vi "Read Settings File.vi"(11 "FIle_Name":string) -> (2 "HV_Voltage_Number":dbl[](array[numeric]), 3 "HV_Voltage_Value_String":string[](array[string]))   [LabVIEW 2013]
uses:
  <vilib>/Utility/file.llb/Read From Spreadsheet File (string).vi
panel:
  out "HV_Settings":string[](array[string])
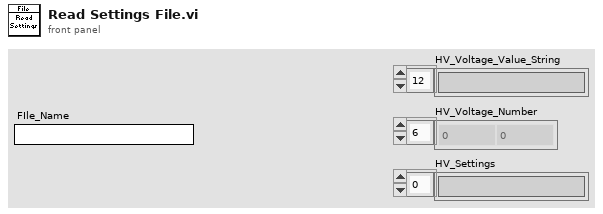
[diagram p1: front panel]
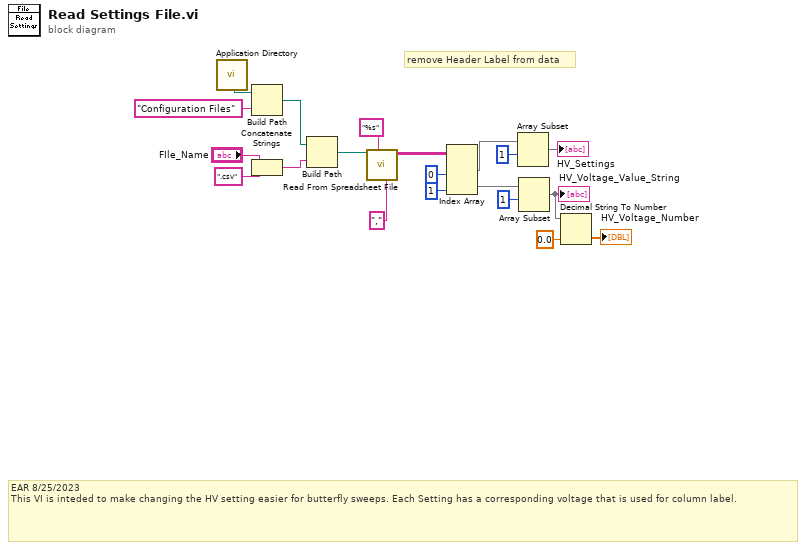
[diagram p0: block diagram]
diagram:
  # "remove Header Label from data"
  # "EAR 8/25/2023\nThis VI is inteded to make changing the HV setting easier for butterfly sweeps. Each Setting has a corresponding voltage that is used for column label."
  n1 = call <vilib>:"Application Directory.vi"() -> ("Application Directory"=w20:path)
  n2 = Build Path(base path=w20, name or relative path="Configuration Files") -> (appended path=w18:path)
  n3 = Concatenate Strings("FIle_Name", ".csv" ("string")) -> (w15:string)
  n4 = Build Path(base path=w18, name or relative path=w15) -> (appended path=w14:path)
  n5 = call-poly <vilib>:"Read From Spreadsheet File.vi"("delimiter (\\t)"="," ("delimiter (\\t)"), "format (%s)"="%s", "file path (dialog if empty)"=w14) -> ("all rows"=w12:string[][])  [unwired: 4 in, 4 out]
  n6 = Index Array(array=w12, index (col) #1=0 ("disabled index (col)"), index (col) #2=1 ("index (col)")) -> (element #1=w7:string[], element #2=w4:string[])  [unwired: 2 in]
  n7 = Array Subset(array=w7, index=1) -> (→"HV_Settings":string[])  [unwired: 1 in]
  n8 = Array Subset(array=w4, index=1) -> (w3:string[])  [unwired: 1 in]
  "HV_Voltage_Value_String" <- w3
  n9 = Decimal String To Number(string=w3, default (0L)=0.0) -> (number=→"HV_Voltage_Number":dbl[])  [unwired: 1 in, 1 out]
